vi "Read dictionary.vi"(8 "error in (no error)":errorcluster, 11 "Config in":refnum<class "Config.lvclass">) -> (0 "error out":errorcluster, 2 "Object RefNum":T1, 3 "Config out":refnum<class "Config.lvclass">)   [LabVIEW 2020, in "Config.lvclass"]
uses:
  Config.lvclass
  <userlib>/_OpenG.lib/dictionary/dictionary.llb/Dictionary Object RefNum__ogtk.ctl
  <userlib>/_OpenG.lib/dictionary/dictionary.llb/Dictionary Object RefNum - Enum__ogtk.ctl
  Config.lvclass/Config.ctl
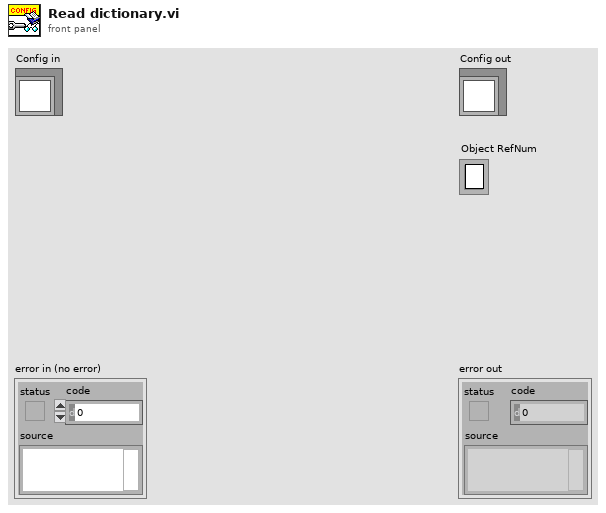
[diagram p1: front panel]
types:
  T1 = typedef "Dictionary Object RefNum__ogtk.ctl" = refnum<k1>
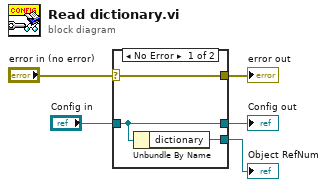
[diagram p0: block diagram]
diagram:
  n1 = case shown="No Error" "error in (no error)" {
    selector: "error in (no error)" -> [w8 w9]
    tunnel: [w8 w9] -> w4
    tunnel: [w6 w10] -> w2
    tunnel: "Config in" -> [w6 w10]
    tunnel: [w7 _] -> w1
    frame No Error {
      n2 = Unbundle By Name(w6) -> ("dictionary"=w7:T1)
    }
    frame Error {
    }
  }
  "error out" <- w4
  "Config out" <- w2
  "Object RefNum" <- w1
